vi "GenerateSineWave.vi"(8 "error in (no error)":errorcluster, 11 "SineModel.lvlib:SineModel.lvclass":refnum<class "SineModel.lvclass">) -> (0 "error out":errorcluster, 3 "SineModel.lvlib:SineModel.lvclass 2":refnum<class "SineModel.lvclass">)   [LabVIEW 2017, in "SineModel.lvlib" / "SineModel.lvclass"]
uses:
  <vilib>/gpm_packages/@cs/example/Dynamic Viewables/SequenceSteps/SineModel/SineModel.lvclass
  C:/Program Files/National Instruments/LabVIEW 2017/vi.lib/gpm_packages/@cs/mva-core/Source/IModel/IModel/IModel.lvclass
  C:/Program Files/National Instruments/LabVIEW 2017/vi.lib/ActorFramework/Actor/Actor.lvclass
  <vilib>/gpm_packages/@cs/example/Dynamic Viewables/SequenceSteps/SineModel/SineModel.lvclass/SineModel.ctl
  <vilib>/gpm_packages/@cs/mva-core/Source/IObserver/IObserver/IObserver.lvclass/IObserver.ctl
  <vilib>/gpm_packages/@cs/mva-core/Source/IModel/IModel/IModel.lvclass/IModel.ctl
  <vilib>/gpm_packages/@cs/mva-core/Source/IMediator/PublishRequest/PublishRequest.lvclass/PublishRequest.ctl
  <vilib>/gpm_packages/@cs/mva-core/Source/IMediator/IMediator Messages/Publish Msg/Publish Msg.lvclass/Publish Msg.ctl
  <vilib>/gpm_packages/@cs/actor-framework-messages/Source/RoundTripMessage/RoundTripMessage.lvclass/RoundTripMessage.ctl
  <vilib>/ActorFramework/Message Enqueuer/Message Enqueuer.lvclass/Message Enqueuer.ctl
  <vilib>/ActorFramework/Actor/Actor.lvclass/Actor.ctl
  cb7bf9b9-956b-4f49-b468-f64f0c203643.vi
  <vilib>/gpm_packages/@cs/mva-core/Source/IMediator/IMediator Messages/Publish Msg/Send Pre-Addressed Publish.vi
  <vilib>/gpm_packages/@cs/mva-core/Source/IObserver/IObserver/Read Unique ID.vi
  <vilib>/gpm_packages/@cs/mva-core/Source/IMediator/PublishRequest/Pack Publish Request.vi
  <vilib>/ActorFramework/Message Enqueuer/Init from Existing Queue.vi
  <vilib>/ActorFramework/Message Enqueuer/Enqueue.vi
  <vilib>/gpm_packages/@cs/actor-framework-messages/Source/RoundTripMessage/Return Round-Trip Message.vi
  <vilib>/gpm_packages/@cs/mva-core/Source/IModel/IModel/IModel.lvclass
  C:/Program Files/National Instruments/LabVIEW 2017/vi.lib/gpm_packages/@cs/mva-core/Source/IObserver/IObserver/IObserver.lvclass
  <vilib>/gpm_packages/@cs/mva-core/Source/IMediator/IMediator Messages/Publish Msg/Publish Msg.lvclass
  C:/Program Files/National Instruments/LabVIEW 2017/vi.lib/gpm_packages/@cs/actor-framework-messages/Source/RoundTripMessage/RoundTripMessage.lvclass
  <vilib>/gpm_packages/@cs/actor-framework-messages/Source/RoundTripMessage/RoundTripMessage.lvclass
  C:/Program Files/National Instruments/LabVIEW 2017/vi.lib/ActorFramework/Message/Message.lvclass
  <vilib>/gpm_packages/@cs/example/Dynamic Viewables/SequenceSteps/SineModel Messages/GenerateSineWave Msg/GenerateSineWave Msg.lvclass
  <vilib>/ActorFramework/Stop Msg/Stop Msg.lvclass
  <vilib>/Utility/error.llb/Error Cluster From Error Code.vi
  <vilib>/ActorFramework/Message Priority Queue/Priority Enqueue.vi
  <vilib>/gpm_packages/@cs/mva-core/Source/IMediator/PublishRequest/PublishRequest.lvclass
  <vilib>/ActorFramework/Message Enqueuer/Message Enqueuer.lvclass
  <vilib>/ActorFramework/Actor/Actor.lvclass
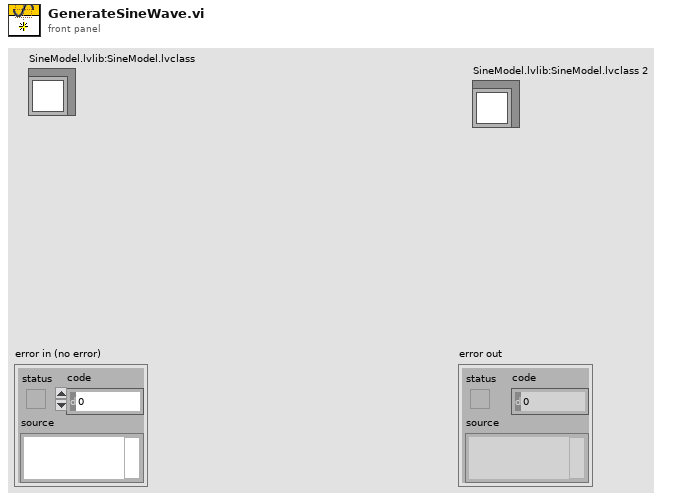
[diagram p1: front panel]
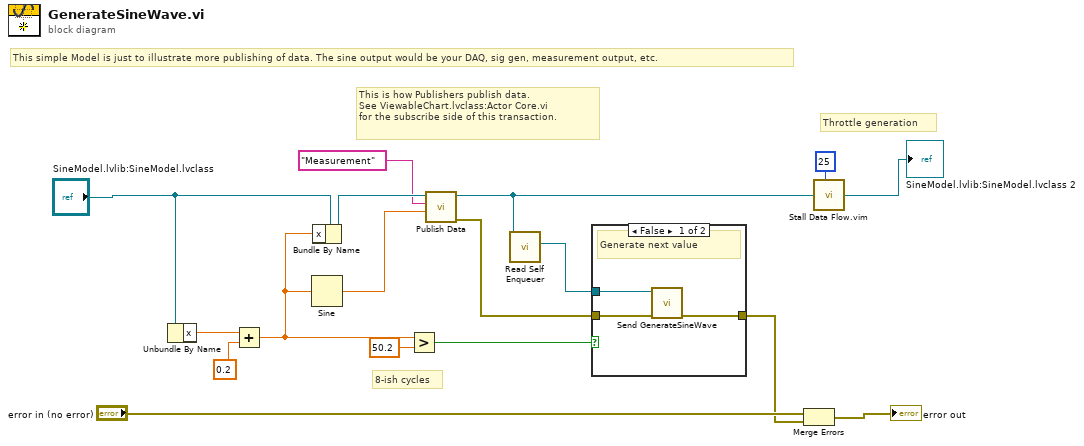
[diagram p0: block diagram]
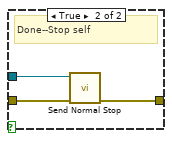
[diagram p2: hidden frame]
diagram:
  # "8-ish cycles"
  # "Throttle generation"
  # "This simple Model is just to illustrate more publishing of data. The sine output would be your DAQ, sig gen, measurement output, etc."
  # "This is how Publishers publish data.\nSee ViewableChart.lvclass:Actor Core.vi\nfor the subscribe side of this transaction."
  n1 = Unbundle By Name("SineModel.lvlib:SineModel.lvclass") -> ("x"=w9:dbl)
  n2 = Add(x=w9, y=0.2) -> (x+y=w5:dbl)
  n3 = Sine(x=w5) -> (sin(x)=w7:dbl)
  n4 = Bundle By Name(cluster="SineModel.lvlib:SineModel.lvclass", "x"=w5) -> (w10:refnum<class "SineModel.lvclass">)
  n5 = Greater?(x=w5, y=50.2) -> (0:w3:bool)
  n6 = call <vilib>:"Publish Data.vi"("Data to Publish"=w7, "Datum Name"="Measurement", "IModel in"=w10) -> ("error out"=w15:errorcluster, "IModel out"=w14:refnum<class "SineModel.lvclass">)  [unwired: 7 in]
  n7 = call <vilib>:"Read Self Enqueuer.vi"("Actor"=w14) -> ("Self Enqueuer"=w13:refnum<class "Message Enqueuer.lvclass">)  [unwired: 10 in]
  n8 = case shown="False" w3 {
    tunnel: w15 -> [w20 w23]
    tunnel: w13 -> [w19 w21]
    tunnel: [w18 w22] -> w12
    frame False {
      # "Generate next value"
      n9 = call <vilib>:"Send GenerateSineWave.vi"("error in (no error)"=w20, "Message Enqueuer"=w19) -> ("error out"=w18:errorcluster)  [unwired: 8 in, 1 out]
    }
    frame True {
      # "Done--Stop self"
      n10 = call <vilib>:"Send Normal Stop.vi"("error in (no error)"=w23, "Message Enqueuer"=w21) -> ("error out"=w22:errorcluster)  [unwired: 9 in]
    }
  }
  n11 = Merge Errors("error in (no error)", w12) -> (→"error out":errorcluster)
  n12 = call "Stall Data Flow.vim"("value in"=w14, "milliseconds to wait"=u32 25) -> ("value out"=→"SineModel.lvlib:SineModel.lvclass 2":refnum<class "SineModel.lvclass">)  [unwired: 1 out]
